vi "CSM - Module VI Reference(with Cache).vi"(6 "Response Timeout(-2 using Global Settings)":i32=-2, 7 "Current Module(\"\" to generate a ID)":string, 8 "error in (no error)":errorcluster, 11 "CSM Name":string) -> (0 "error out":errorcluster, 3 "CSM Module VIRef":refnum<vi>)   [LabVIEW 2017, in "CSM-Helper API with lvcsm Support.lvlib"]
uses:
  CSM-Helper API with lvcsm Support.lvlib
  Communicable State Machine.lvlib
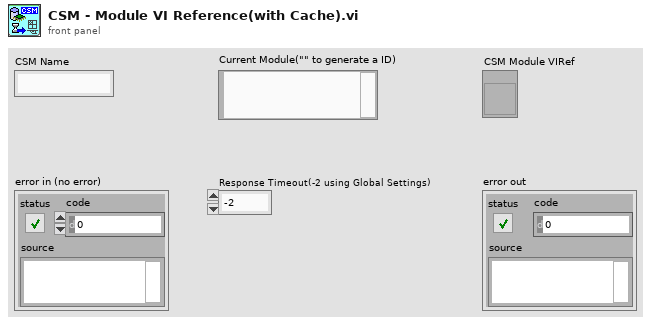
[diagram p1: front panel]
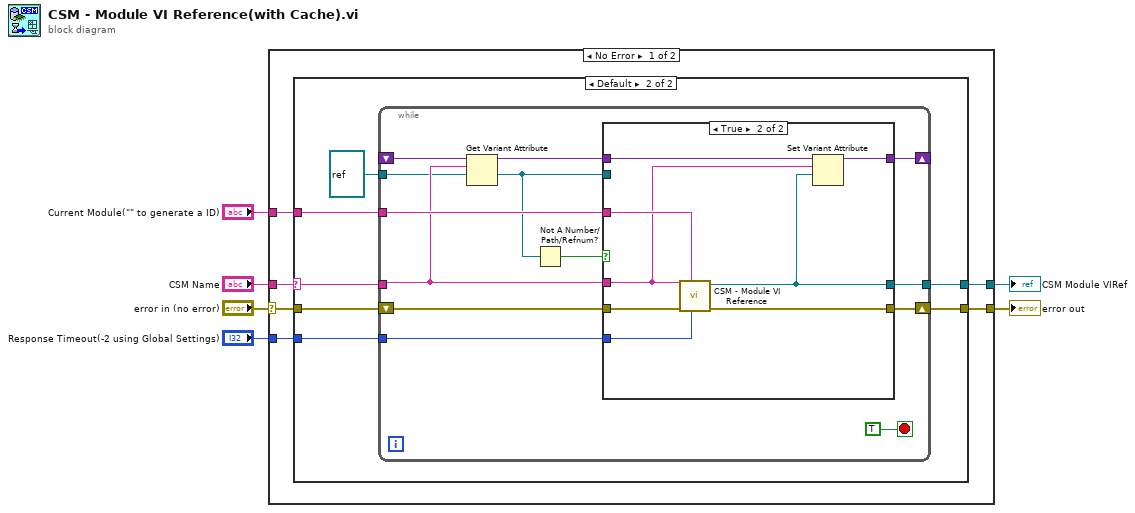
[diagram p0: block diagram]
diagram:
  n1 = case shown="No Error" "error in (no error)" {
    selector: "error in (no error)" -> [w10 w45]
    tunnel: "Response Timeout(-2 using Global Settings)" -> [w12 _]
    tunnel: "Current Module(\"\" to generate a ID)" -> [w11 _]
    tunnel: "CSM Name" -> [w9 _]
    tunnel: [w8 w45] -> w2
    tunnel: [w7 _] -> w1
    frame No Error {
      n2 = case shown="Default" w9 {
        selector: w9 -> [_ w17]
        tunnel: w12 -> [_ w20]
        tunnel: w11 -> [_ w19]
        tunnel: w10 -> [w13 w18]
        tunnel: [w13 w16] -> w8
        tunnel: [_ w15] -> w7
        frame "" {
        }
        frame Default {
          n3 = while {
            tunnel: w20 -> [w33]
            tunnel: w19 -> [w32]
            tunnel: w17 -> [w26]
            tunnel: [w29] -> w15
            shift-right: [w30] -> w16
            shift-left: w18 -> [w31]
            shift-right: [w23] -> _
            shift-left: _ -> [w27]
            tunnel: refnum<vi> refnum ("CSM Module VIRef") -> [w25]
            stop <- TRUE stop-if-true
            n4 = Get Variant Attribute(Variant=w27, name=w26, default value (empty Variant)=w25) -> (duplicate Variant=w22:variant, value=w21:refnum<vi>)  [unwired: 1 in, 2 out]
            n5 = Not A Number/Path/Refnum?(number/path/refnum=w21) -> (NaN/Path/Refnum?=w24:bool)
            n6 = case shown="True" w24 {
              tunnel: w33 -> [_ w44]
              tunnel: w32 -> [_ w43]
              tunnel: w31 -> [w34 w42]
              tunnel: [w34 w41] -> w30
              tunnel: [w35 w37] -> w29
              tunnel: w26 -> [_ w38]
              tunnel: [w36 w39] -> w23
              tunnel: w22 -> [w36 w40]
              tunnel: w21 -> [w35 _]
              frame False {
              }
              frame True {
                n7 = call "CSM - Module VI Reference.vi"("Response Timeout(-2 using Global Settings)"=w44, "Current Module(\"\" to generate a ID)"=w43, "error in (no error)"=w42, "CSM Name"=w38) -> ("error out"=w41:errorcluster, "CSM Module VIRef"=w37:refnum<vi>)  [unwired: 6 in]
                n8 = Set Variant Attribute(Variant=w40, name=w38, value=w37) -> (Variant out=w39:variant)  [unwired: 1 in, 2 out]
              }
            }
          }
        }
      }
    }
    frame Error {
    }
  }
  "error out" <- w2
  "CSM Module VIRef" <- w1
